vi "二分法-单数值插入一维数组位置输出.vi"(8 "数值":dbl format="%#_13g", 11 "一维数组":dbl[](array[numeric])) -> (0 "错误输出":errorcluster caption="错误常量", 2 "插入此索引处":i32, 3 "最近索引":i32)   [LabVIEW 2017]
panel:
  out "s? t:f":enum16{"从小到大", "从大到小"}(ring)
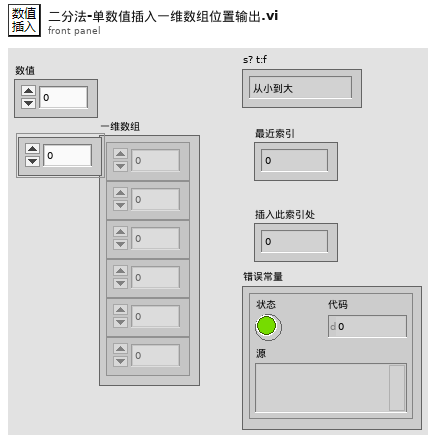
[diagram p1: front panel]
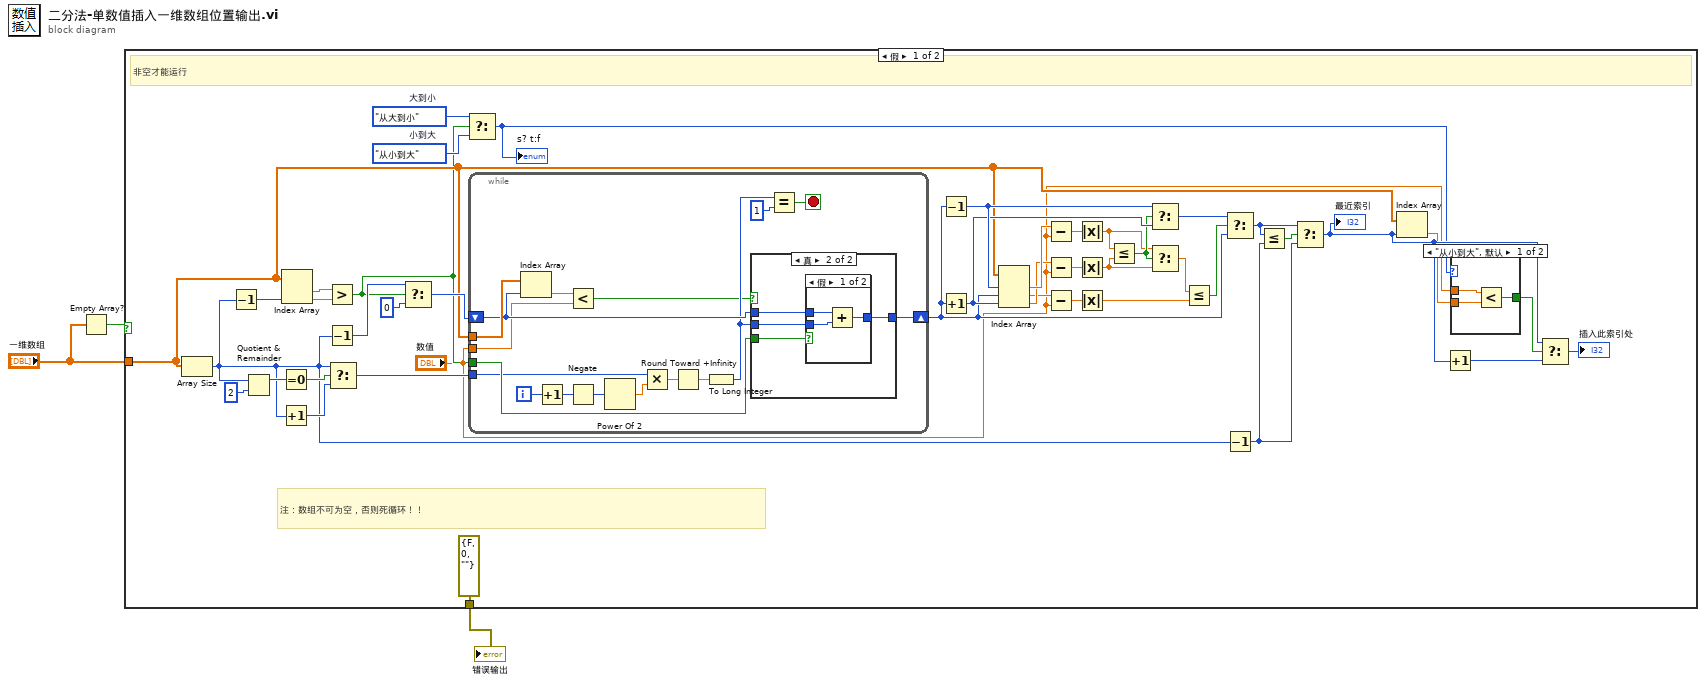
[diagram p0: block diagram]
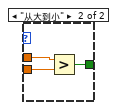
[diagram p2: hidden frame]
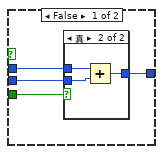
[diagram p3: hidden frame]
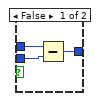
[diagram p4: hidden frame]
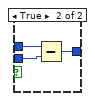
[diagram p5: hidden frame]
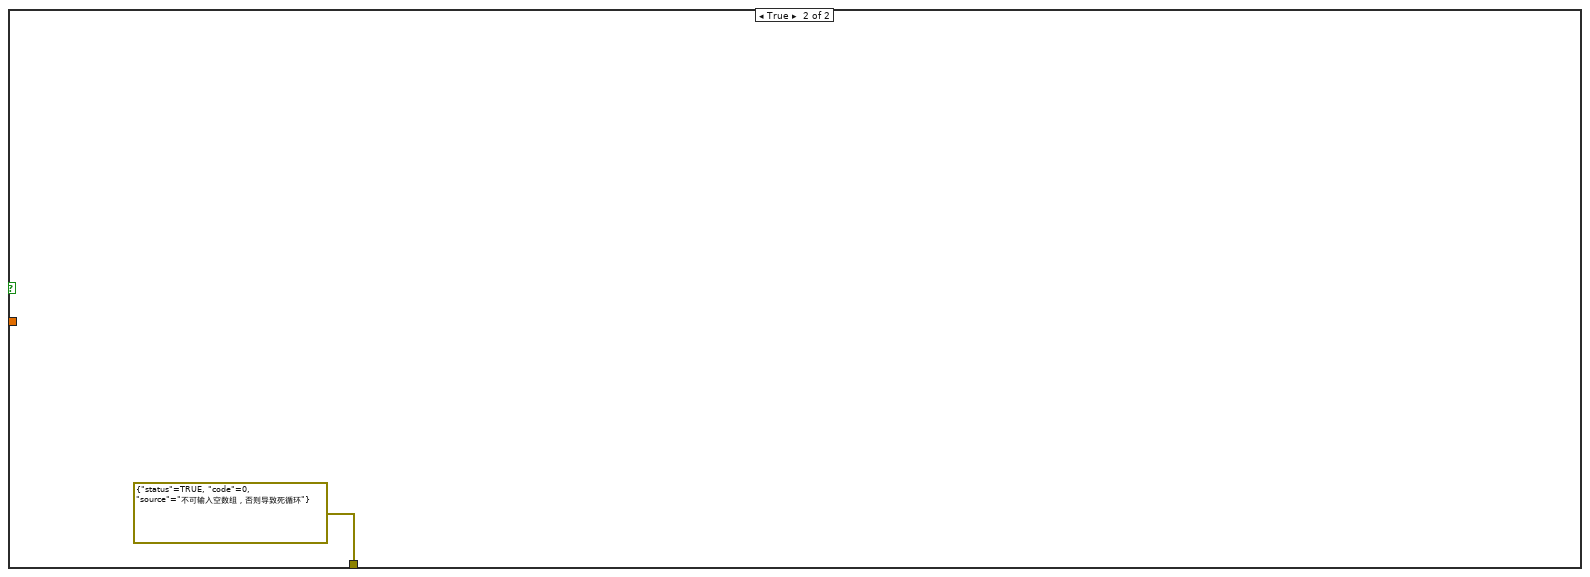
[diagram p6: hidden frame]
diagram:
  n1 = Empty Array?(array="一维数组") -> (empty?=w2:bool)
  n2 = case shown="假" w2 {
    tunnel: "一维数组" -> [w18 _]
    tunnel: [errorcluster {"status"=FALSE, "code"=0, "source"=""} ("错误常量") errorcluster {"status"=TRUE, "code"=0, "source"="不可输入空数组，否则导致死循环"} ("错误常量")] -> w1
    frame False {
      w23 = enum16{"从小到大", "从大到小"}."从小到大"  # 小到大
      w24 = enum16{"从小到大", "从大到小"}."从大到小"  # 大到小
      # "注：数组不可为空，否则死循环！！"
      # "非空才能运行"
      n3 = Array Size(array=w18) -> (size(s)=w19:i32)
      n4 = Decrement(x=w19) -> (x-1=w46:i32)
      n5 = Quotient & Remainder(x=w19, y=2) -> (x-y*floor(x/y)=w44:i32)  [unwired: 1 out]
      n6 = Equal To 0?(x=w44) -> (x = 0?=w43:bool)
      n7 = Increment(x=w19) -> (x+1=w42:i32)
      n8 = Index Array(array=w18, index #2=w46) -> (element #1=w16:dbl, element #2=w15:dbl)  [unwired: 1 in]
      n9 = Greater?(x=w16, y=w15) -> (0:w17:bool)
      n10 = Decrement(x=w19) -> (x-1=w27:i32)
      n11 = Select(t=w19, s=w43, f=w42) -> (s? t:f=w41:i32)
      n12 = Select(t=w27, s=w17, f=0 ("索引")) -> (s? t:f=w25:i32)
      n13 = Select(t=w24, s=w17, f=w23) -> (s? t:f=w8:enum16{"从小到大", "从大到小"})
      "s? t:f" <- w8
      n14 = while {
        tunnel: w18 -> [w69]
        tunnel: "数值" -> [w53]
        shift-right: [w65] -> w29
        shift-left: w25 -> [w66]
        tunnel: w41 -> [w58]
        tunnel: w17 -> [w68]
        i -> [w61]
        stop <- w62 stop-if-true
        n15 = Index Array(array=w69, index=w66) -> (element=w54:dbl)
        n16 = Increment(x=w61) -> (x+1=w60:i32)
        n17 = Less?(x=w54, y=w53) -> (x < y?=w55:bool)
        n18 = Negate(x=w60) -> (-x=w59:i32)
        n19 = Power Of 2(x=w59) -> (2^x=w57:dbl)
        n20 = Multiply(x=w58, y=w57) -> (x*y=w56:dbl)
        n21 = Round Toward +Infinity(x=w56) -> (ceil(x): smallest int >= x=w67:dbl)
        n22 = To Long Integer(number=w67) -> (32bit integer=w64:i32)
        n23 = case shown="真" w55 {
          tunnel: w68 -> [w73 w83]
          tunnel: w64 -> [w72 w82]
          tunnel: w66 -> [w71 w81]
          tunnel: [w70 w80] -> w65
          frame False {
            n24 = case shown="真" w73 {
              tunnel: w72 -> [w76 w79]
              tunnel: w71 -> [w75 w78]
              tunnel: [w74 w77] -> w70
              frame False {
                n25 = Subtract(x=w75, y=w76) -> (x-y=w74:i32)
              }
              frame True {
                n26 = Add(x=w78, y=w79) -> (x+y=w77:i32)
              }
            }
          }
          frame True {
            n27 = case shown="假" w83 {
              tunnel: w82 -> [w86 w89]
              tunnel: w81 -> [w85 w88]
              tunnel: [w84 w87] -> w80
              frame False {
                n28 = Add(x=w85, y=w86) -> (x+y=w84:i32)
              }
              frame True {
                n29 = Subtract(x=w88, y=w89) -> (x-y=w87:i32)
              }
            }
          }
        }
        n30 = Equal?(x=w64, y=1) -> (x = y?=w62:bool)
      }
      n31 = Decrement(x=w29) -> (x-1=w32:i32)
      n32 = Increment(x=w29) -> (x+1=w31:i32)
      n33 = Index Array(array=w18, index #1=w32, index #2=w29, index #3=w31) -> (element #1=w40:dbl, element #2=w33:dbl, element #3=w35:dbl)
      n34 = Subtract(x=w40, y="数值") -> (x-y=w38:dbl)
      n35 = Subtract(x=w35, y="数值") -> (x-y=w39:dbl)
      n36 = Subtract(x=w33, y="数值") -> (x-y=w34:dbl)
      n37 = Absolute Value(x=w38) -> (abs(x)=w13:dbl)
      n38 = Absolute Value(x=w39) -> (abs(x)=w12:dbl)
      n39 = Absolute Value(x=w34) -> (abs(x)=w9:dbl)
      n40 = Less Or Equal?(x=w13, y=w12) -> (x <= y?=w14:bool)
      n41 = Select(t=w32, s=w14, f=w31) -> (s? t:f=w30:i32)
      n42 = Select(t=w13, s=w14, f=w12) -> (s? t:f=w10:dbl)
      n43 = Less Or Equal?(x=w10, y=w9) -> (x <= y?=w11:bool)
      n44 = Select(t=w30, s=w11, f=w29) -> (s? t:f=w28:i32)
      n45 = Decrement(x=w19) -> (x-1=w36:i32)
      n46 = Less Or Equal?(x=w28, y=w36) -> (x <= y?=w37:bool)
      n47 = Select(t=w28, s=w37, f=w36) -> (s? t:f=w22:i32)
      "最近索引" <- w22
      n48 = Index Array(array=w18, index=w22) -> (element=w6:dbl)
      n49 = Increment(x=w22) -> (x+1=w21:i32)
      n50 = case shown="\"从小到大\", 默认" w8 {
        tunnel: [w49 w52] -> w5
        tunnel: "数值" -> [w48 w51]
        tunnel: w6 -> [w47 w50]
        frame "从小到大", Default {
          n51 = Less?(x=w48, y=w47) -> (x < y?=w49:bool)
        }
        frame "从大到小" {
          n52 = Greater?(x=w51, y=w50) -> (0:w52:bool)
        }
      }
      n53 = Select(t=w22, s=w5, f=w21) -> (s? t:f=→"插入此索引处":i32)
    }
    frame True {
    }
  }
  "错误输出" <- w1
